vi "1D Quadrature (VI).vi"(7 "data":variant, 8 "tolerance":dbl=1e-05, 9 "lower limit":dbl, 10 "upper limit":dbl=1.0, 11 "integrand":refnum<vi>) -> (0 "error":i32, 3 "result":dbl)   [LabVIEW 2014, in "NI_AALPro.lvlib"]
doc: "Performs numerical integration using adaptive quadrature approach. You must manually select the polymorphic instance to use."
uses:
  NI_AALPro.lvlib
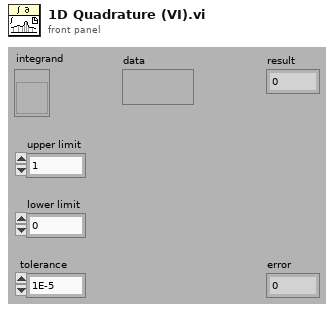
[diagram p1: front panel]
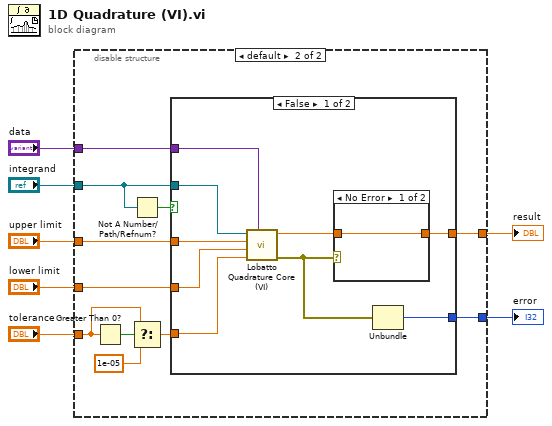
[diagram p0: block diagram]
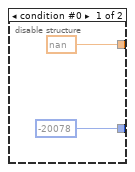
[diagram p2: hidden frame]
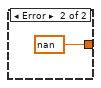
[diagram p3: hidden frame]
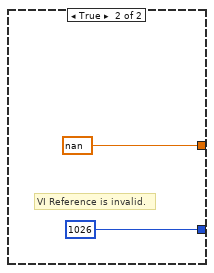
[diagram p4: hidden frame]
diagram:
  n1 = disable-structure shown="default" {
    disable-tunnel: [-20078 ("code") w20] -> w7
    disable-tunnel: "upper limit" -> [_ w19]
    disable-tunnel: "lower limit" -> [_ w18]
    disable-tunnel: "tolerance" -> [_ w11]
    disable-tunnel: [nan ("result") w17] -> w3
    disable-tunnel: "integrand" -> [_ w15]
    disable-tunnel: "data" -> [_ w14]
    frame condition #0 {
    }
    frame condition #1 (active) {
      n2 = Greater Than 0?(x=w11) -> (x > 0?=w13:bool)
      n3 = Not A Number/Path/Refnum?(number/path/refnum=w15) -> (NaN/Path/Refnum?=w16:bool)
      n4 = Select(t=w11, s=w13, f=1e-05) -> (s? t:f=w12:dbl)
      n5 = case shown="False" w16 {
        tunnel: [w29 nan] -> w17
        tunnel: [w28 1026] -> w20
        tunnel: w19 -> [w27 _]
        tunnel: w18 -> [w26 _]
        tunnel: w12 -> [w25 _]
        tunnel: w15 -> [w24 _]
        tunnel: w14 -> [w23 _]
        frame False {
          n6 = call "Lobatto Quadrature Core (VI).vi"("data"=w23, "tolerance"=w25, "lower limit"=w26, "upper limit"=w27, "f(x)"=w24) -> ("error out"=w21:errorcluster, "result"=w22:dbl)  [unwired: 5 out]
          n7 = case shown="No Error" w21 {
            tunnel: w22 -> [w30 _]
            tunnel: [w30 nan] -> w29
            frame No Error {
            }
            frame Error {
            }
          }
          n8 = Unbundle(w21) -> ("code"=w28:i32)  [unwired: 2 out]
        }
        frame True {
          # "VI Reference is invalid."
        }
      }
    }
  }
  "error" <- w7
  "result" <- w3
